vi "Apply.vi"(8 "error in (no error)":errorcluster, 11 "FGen PXI Std Waveform CFG in":refnum<class "FGen PXI Std Waveform CFG.lvclass">) -> (0 "error out":errorcluster, 3 "FGen PXI Std Waveform CFG out":refnum<class "FGen PXI Std Waveform CFG.lvclass">)   [LabVIEW 2023, in "FGen PXI Std Waveform CFG.lvlib" / "FGen PXI Std Waveform CFG.lvclass"]
uses:
  FGen PXI Std Waveform CFG.lvclass
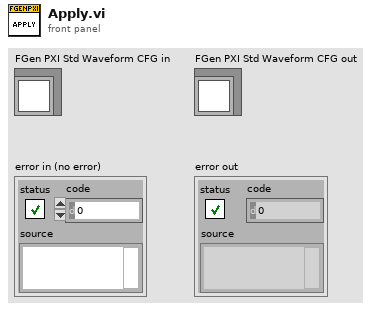
[diagram p1: front panel]
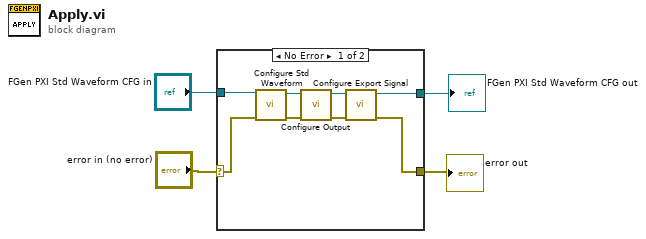
[diagram p0: block diagram]
diagram:
  n1 = case shown="No Error" "error in (no error)" {
    selector: "error in (no error)" -> [w11 w14]
    tunnel: "FGen PXI Std Waveform CFG in" -> [w12 w13]
    tunnel: [w8 w13] -> w2
    tunnel: [w9 w14] -> w1
    frame No Error {
      n2 = call-dynamic "Configure Std Waveform.vi"("error in (no error)"=w11, "FGen PXI Base CFG in"=w12) -> ("error out"=w10:errorcluster, "FGen PXI Base CFG out"=w6:refnum<class "FGen PXI Std Waveform CFG.lvclass">)  [unwired: 8 in]
      n3 = call-dynamic "Configure Output.vi"("error in (no error)"=w10, "FGen PXI Base CFG in"=w6) -> ("error out"=w7:errorcluster, "FGen PXI Base CFG out"=w5:refnum<class "FGen PXI Std Waveform CFG.lvclass">)  [unwired: 8 in]
      n4 = call-dynamic "Configure Export Signal.vi"("error in (no error)"=w7, "FGen PXI Base CFG in"=w5) -> ("error out"=w9:errorcluster, "FGen PXI Base CFG out"=w8:refnum<class "FGen PXI Std Waveform CFG.lvclass">)  [unwired: 8 in]
    }
    frame Error {
    }
  }
  "error out" <- w1
  "FGen PXI Std Waveform CFG out" <- w2
